vi "测试-读取摄像头.vi"() -> ()   [LabVIEW 2018]
uses:
  <vilib>/userdefined/High Color/IMAQdx.ctl
  <vilib>/vision/driver/NI_Vision_Acquisition_Software.lvlib
panel:
  out "读取帧率fps":dbl
  out "图片保存路径":path
  in  "保存图片名":string
  in  "IMAQdx Session":T1
  in  "关闭程序":bool
  out "?":T2(plugin-control)
  in  "拍照":bool
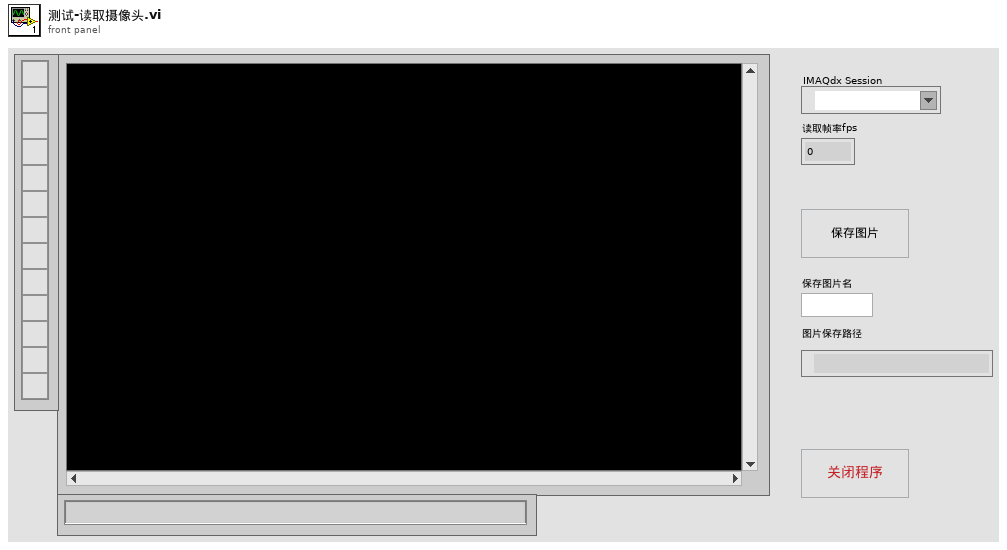
[diagram p1: front panel]
types:
  T1 = typedef "IMAQdx.ctl" = refnum<k21>
  T2 = typedef "IMAQ Image.ctl" = refnum<image>
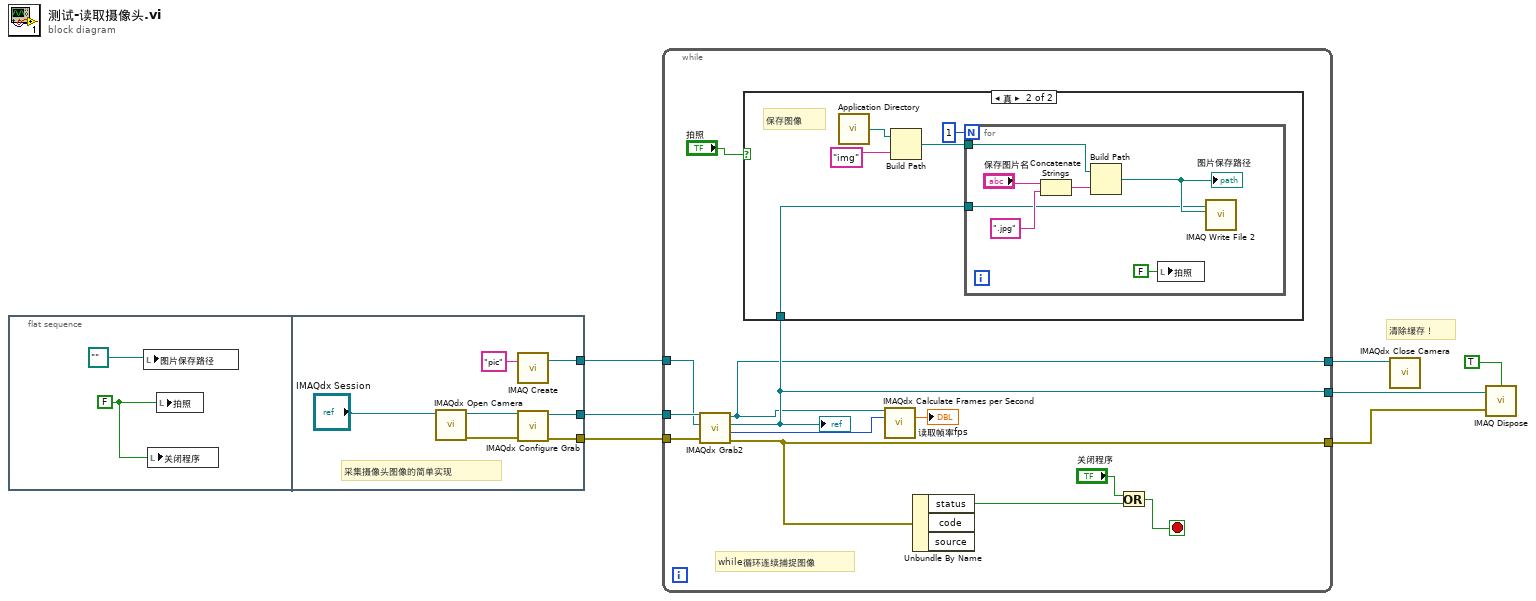
[diagram p0: block diagram]
diagram:
  # "清除缓存！"
  n1 = flat-sequence {
    tunnel: [w12] -> w3
    tunnel: [w11] -> w2
    tunnel: [w10] -> w1
    frame #0 {
      w9 = FALSE ("拍照")
      n2 = local write "图片保存路径"(path "" ("图片保存路径")) -> ()
      n3 = local write "关闭程序"(w9) -> ()
      n4 = local write "拍照"(w9) -> ()
    }
    frame #1 {
      # "采集摄像头图像的简单实现"
      n5 = call <vilib>:"IMAQdx Open Camera.vi"("Session In"="IMAQdx Session") -> ("error out"=w16:errorcluster, "Session Out"=w15:T1)  [unwired: 9 in]
      n6 = call "IMAQ Create"("Image Name"="pic") -> ("New Image"=w12:T2)  [unwired: 4 in, 1 out]
      n7 = call <vilib>:"IMAQdx Configure Grab.vi"("error in"=w16, "Session In"=w15) -> ("error out"=w11:errorcluster, "Session Out"=w10:T1)  [unwired: 8 in]
    }
  }
  n8 = while {
    tunnel: w1 -> [w28]
    tunnel: w3 -> [w27]
    tunnel: [w21] -> w7
    tunnel: [w18] -> w6
    tunnel: w2 -> [w26]
    tunnel: [w22] -> w5
    stop <- w23 stop-if-true
    # "while循环连续捕捉图像"
    n9 = call <vilib>:"IMAQdx Grab2.vi"("error in"=w26, "Image In"=w27, "Session In"=w28) -> ("error out"=w22:errorcluster, "Buffer Number Out"=w20:u32, "Image Out"=w21:T2, "Session Out"=w18:T1)  [unwired: 5 in]
    "?" <- w21
    n10 = case shown="真" "拍照" {
      tunnel: w21 -> [_ w31]
      frame False {
      }
      frame True {
        # "保存图像"
        n11 = call <vilib>:"Application Directory.vi"() -> ("Application Directory"=w33:path)
        n12 = Build Path(base path=w33, name or relative path="img" ("名称或相对路径")) -> (appended path=w32:path)
        n13 = for {
          N: 1 -> [_]
          tunnel: w32 -> [w38]
          tunnel: w31 -> [w36]
          n14 = Concatenate Strings("保存图片名", ".jpg" ("名称或相对路径")) -> (w40:string)
          n15 = Build Path(base path=w38, name or relative path=w40) -> (appended path=w37:path)
          "图片保存路径" <- w37
          n16 = local write "拍照"(FALSE ("拍照")) -> ()
          n17 = call-poly "IMAQ Write File 2"("File Path"=w37, "Image"=w36) -> ()  [unwired: 8 in, 2 out]
        }
      }
    }
    n18 = call <vilib>:"IMAQdx Calculate Frames per Second.vi"("Session In"=w18, "Buffer Number"=w20) -> ("Acquired Frames per Second"=→"读取帧率fps":dbl)  [unwired: 7 in, 6 out]
    n19 = Unbundle By Name(w22) -> ("status"=w24:bool)  [unwired: 2 out]
    n20 = Or(x="关闭程序", y=w24) -> (x .or. y?=w23:bool)
  }
  n21 = call <vilib>:"IMAQdx Close Camera.vi"("Session In"=w6) -> ()  [unwired: 10 in, 1 out]
  n22 = call "IMAQ Dispose"("All Images? (No)"=TRUE, "Image"=w7, "error in (no error)"=w5) -> ()  [unwired: 3 in, 1 out]
